vi "VDMS_NO_IEPE_FPGA_Main_6_Modules.vi"() -> ()   [LabVIEW 2017]
doc: "This VI provides a template for customizing a waveform acquisition using delta-sigma based NI C Series analog input smodules."
uses:
  <vilib>/LabVIEW Targets/FPGA/cRIO/shared/nicrio_ModuleControls/nicrio_cRIO-9232_ConfigModeRing.ctl
  <vilib>/Platform/TimedLoop/XDataNode/timing_clust.ctl
  <vilib>/Platform/TimedLoop/XDataNode/nitl_modes.ctl
  <vilib>/Platform/TimedLoop/XDataNode/wakeup.ctl
  <vilib>/rvi/Emulation/niFpgaGetClockAttributes.vi
  <vilib>/rvi/Emulation/niFpgaSctlEmulationGetInTimedLoop.vi
  <vilib>/rvi/Emulation/niFpgaEmulationReportErrorSimple.vi
  <vilib>/rvi/Emulation/niFpgaProcessEmulError.vi
  <vilib>/addons/InsightCM/Devices/Shared/Cms/Fpga/AcquisitionFpgaTach/source/subVIs/Glbl Stop.vi
  <vilib>/addons/InsightCM/Devices/Shared/Cms/Fpga/AcquisitionFpgaTach/source/subVIs/FPGA Globals.vi
  <vilib>/rvi/eio/common/nirviEmuTemplateMethod_errors.vi
  <vilib>/rvi/Memory/Memory_Emulation/nirvimemoryFastEmulation.vi
  <vilib>/rvi/Memory/Memory_Emulation/nirvimemoryEmulation.vi
  <vilib>/rvi/Emulation/niFpgaEmulationIsFPGAContextNoSignature.vi
  <vilib>/rvi/DataTransferAndStorage/Container/Common/niFpgaContainerGetUniqueNameForEmu.vi
  <vilib>/rvi/errors/nirviReportUnexpectedCaseInternalError (U32).vi
  <vilib>/rvi/DataTransferAndStorage/Container/Common/niFpgaContainerExecOnDevCompGetState.vi
  <vilib>/rvi/Memory/Memory_Emulation/niFpgaMemoryEmulationCacheClearOnFirstRun.vi
  <vilib>/rvi/Memory/Memory_Emulation/nirvimemoryEmulationManagerCache_MakeExclusive.vi
  <vilib>/rvi/Memory/Memory_Emulation/niFpgaMemoryEmulationValidateCache.vi
  <vilib>/rvi/Memory/Memory_Emulation/nirvimemoryEmulationManagerCache_InsertValue.vi
  <vilib>/Utility/error.llb/Clear Errors.vi
  <vilib>/rvi/Memory/Memory_Emulation/nirvimemoryEmulationManagerCache_ReleaseExclusive.vi
  <vilib>/rvi/Memory/Memory_Emulation/nirvimemoryEmulationManagerCache_GetValue.vi
  <vilib>/rvi/Memory/Memory_Emulation/nirvimemoryEmulationManagerCache_SetValue.vi
  <vilib>/rvi/Emulation/niFpgaSctlEmulationResourceMgr.vi
  <vilib>/rvi/Emulation/niFpgaCriticalErrorInLSC.vi
  <vilib>/rvi/interface/RandomDataEmulation/niFpgaRandomDataHandleErrors.vi
  <vilib>/rvi/errors/niFpgaSetErrorForExecOnDevCompSimple.vi
  <vilib>/rvi/eio/common/nirviEmuReportErrorAndStop.vi
  <vilib>/rvi/FIFO/Fifo_Resource/nirvififoEmulationSetSize.vi
  <vilib>/rvi/FIFO/Fifo_Resource/nirviFifoEmulationQueueMgr.vi
  <instcachedir>/0/nirviFifoEmulationQueueMgr_E5CAEC123FF24DC58D834DCA3CDAA9B5.lvgen/nirviFifoEmulationQueueMgr_E5CAEC123FF24DC58D834DCA3CDAA9B5_001.vi
  <vilib>/rvi/FIFO/Fifo_Resource/nirvififoEmulationDetermineInputValidOut.vi
  <vilib>/rvi/FIFO/Fifo_Resource/nirvififoEmulationCreateLock.vi
  <vilib>/rvi/FIFO/Fifo_Resource/nirvififoEmulationObtainLock.vi
  <vilib>/rvi/FIFO/Fifo_Resource/nirvififoEmulationReleaseLock.vi
  <vilib>/rvi/occurrence/nirviWaitOnOccurrenceBase.vi
  <vilib>/rvi/errors/nirviReportUnexpectedCaseInternalError.vi
  <vilib>/eio/EIONode/EIONode.xnode
  <vilib>/rvi/DataTransferAndStorage/Container/XNode/niFpgaContainer.xnode
  <vilib>/rvi/Memory/Memory_Emulation/niFpgaMemoryEmulationRefIn.vi
  <vilib>/Platform/TimedLoop/XDataNode/XDataNode.xnode
  <vilib>/rvi/interface/RandomDataEmulation/nirviRandomDataFpgaReadWriteTemplate.vi
  <vilib>/rvi/FXPMathLib/basic elements/FxpDiscreteDelay/XNode/nifxpmath_DiscreteDelay.xnode
  <vilib>/rvi/FIFO/Fifo_Resource/niFpgaFifoEmulationRefIn.vi
  <vilib>/addons/InsightCM/Devices/Shared/Cms/Fpga/AcquisitionFpgaTach/source/subVIs/VibAPI/VDMS_VibAPI.lvlib
  <vilib>/Platform/TimedLoop/XDataNode/XDNodeRunTimeDep.lvlib
panel:
  in  "Tach Delay":u8
  out "Chassis Temperature":sgl
  in  "Enable Chan Array":bool[](array[boolean])=[FALSE, FALSE, FALSE, FALSE, FALSE, FALSE, FALSE, FALSE, FALSE, FALSE, FALSE, FALSE, FALSE, FALSE, FALSE, FALSE, FALSE, FALSE, FALSE, FALSE, FALSE, FALSE, FALSE, FALSE]
  in  "Custom Scale Intercept":sgl[](array[numeric])=[0.0, 0.0, 0.0, 0.0, 0.0, 0.0, 0.0, 0.0, 0.0, 0.0, 0.0, 0.0, 0.0, 0.0, 0.0, 0.0, 0.0, 0.0, 0.0, 0.0, 0.0, 0.0, 0.0, 0.0]
  in  "Custom Scale Slope":sgl[](array[numeric])=[0.0, 0.0, 0.0, 0.0, 0.0, 0.0, 0.0, 0.0, 0.0, 0.0, 0.0, 0.0, 0.0, 0.0, 0.0, 0.0, 0.0, 0.0, 0.0, 0.0, 0.0, 0.0, 0.0, 0.0]
  in  "Threshold2":fxp<+/-,24,7>=-10.0
  in  "Slope2":enum16{"falling", "rising"}(ring)
  in  "Hysteresis2":fxp<+/-,24,7>=1.0
  in  "Hysteresis1":fxp<+/-,24,7>=1.0
  in  "Threshold1":fxp<+/-,24,7>=-10.0
  in  "Slope1":enum16{"falling", "rising"}(ring)
  in  "Hysteresis0":fxp<+/-,24,7>=1.0
  in  "Slope0":enum16{"falling", "rising"}(ring)
  in  "Threshold0":fxp<+/-,24,7>=-10.0
  out "Tach FIFO Full":bool
  in  "Delay Comp":u32
  out "Start Trigger":bool
  in  "Number of Modules":i16=1
  out "Open Loop Chan Array":bool[](array[boolean])
  out "Short Circuit Chan Array":bool[](array[boolean])
  in  "Input Config Array":T1[](array[typedef])=[1, 1, 1, 1, 1, 1, 1, 1, 1, 1, 1, 1, 1, 1, 1, 1, 1, 1, 1, 1, 1, 1, 1, 1] items=["AC Coupled", "DC Coupled", "IEPE AC Coupled"]
  in  "Data Rate [S/s]":u32=1280
  out "Chan Count":bool
  out "Acq Loop Ticks":u32
  out "FPGA Error":errorcluster
  out "Module Underflow":bool
  out "Finished":bool
  in  "Total Avail Channels":i32=4
  in  "Samps per Chan [Finite]":i32=5120
  out "First Read":bool
  in  "Acquisition Type":enum16{"Finite Samples", "Continuous Samples"}(ring)
  out "DMA FIFO Full":bool
  in  "Stop":bool
  # "Keyphasor Info"
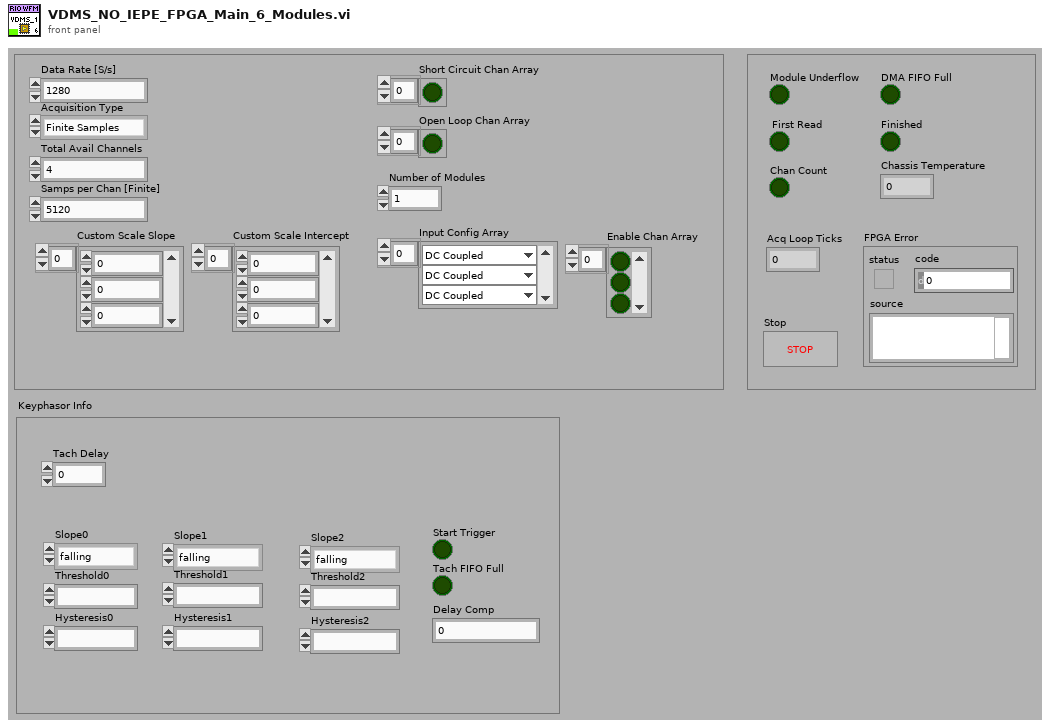
[diagram p1: front panel]
types:
  T1 = typedef "nicrio_cRIO-9232_ConfigModeRing.ctl" = u8
  T2 = typedef "XDNodeRunTimeDep.lvlib/timing_clust.ctl" = cluster{"Expected End [f-1]":u64, "Actual End [f-1]":u64, "Finished Late? [f-1]":bool, "Expected End [i-1]":u64, "Actual End [i-1]":u64, "Finished Late? [i-1]":bool, "Expected Start [i]":u64, "Actual Start [i]":u64, "Expected Start [f]":u64, "Actual Start [f]":u64, "Source Name":string, "Structure Name":string, "Period":i64, "Deadline":i64, "Offset":i64, "Start":i64, "Priority":i32, "Timeout":i32, "Mode":T3, "Wakeup Reason":T4, "Error":errorcluster, "Source Type":string, "Secondary Source Type":string, "Global End Time":u64, "Global Start Time":u64, "Frame Duration":u64, "Iteration Duration":u64, "Assigned CPU":i32, "I/O Scan Engine Mode":u32}
  T3 = typedef "XDNodeRunTimeDep.lvlib/nitl_modes.ctl" = enum32{"No Change", "Process missed periods, maintain original phase", "Discard missed periods, maintain original phase", "Process missed periods, ignore original phase", "Discard missed periods, ignore original phase"}
  T4 = typedef "XDNodeRunTimeDep.lvlib/wakeup.ctl" = enum32{"Normal", "Aborted", "Asynchronous wakeup", "Timing source error", "Timed loop error", "Timeout"}
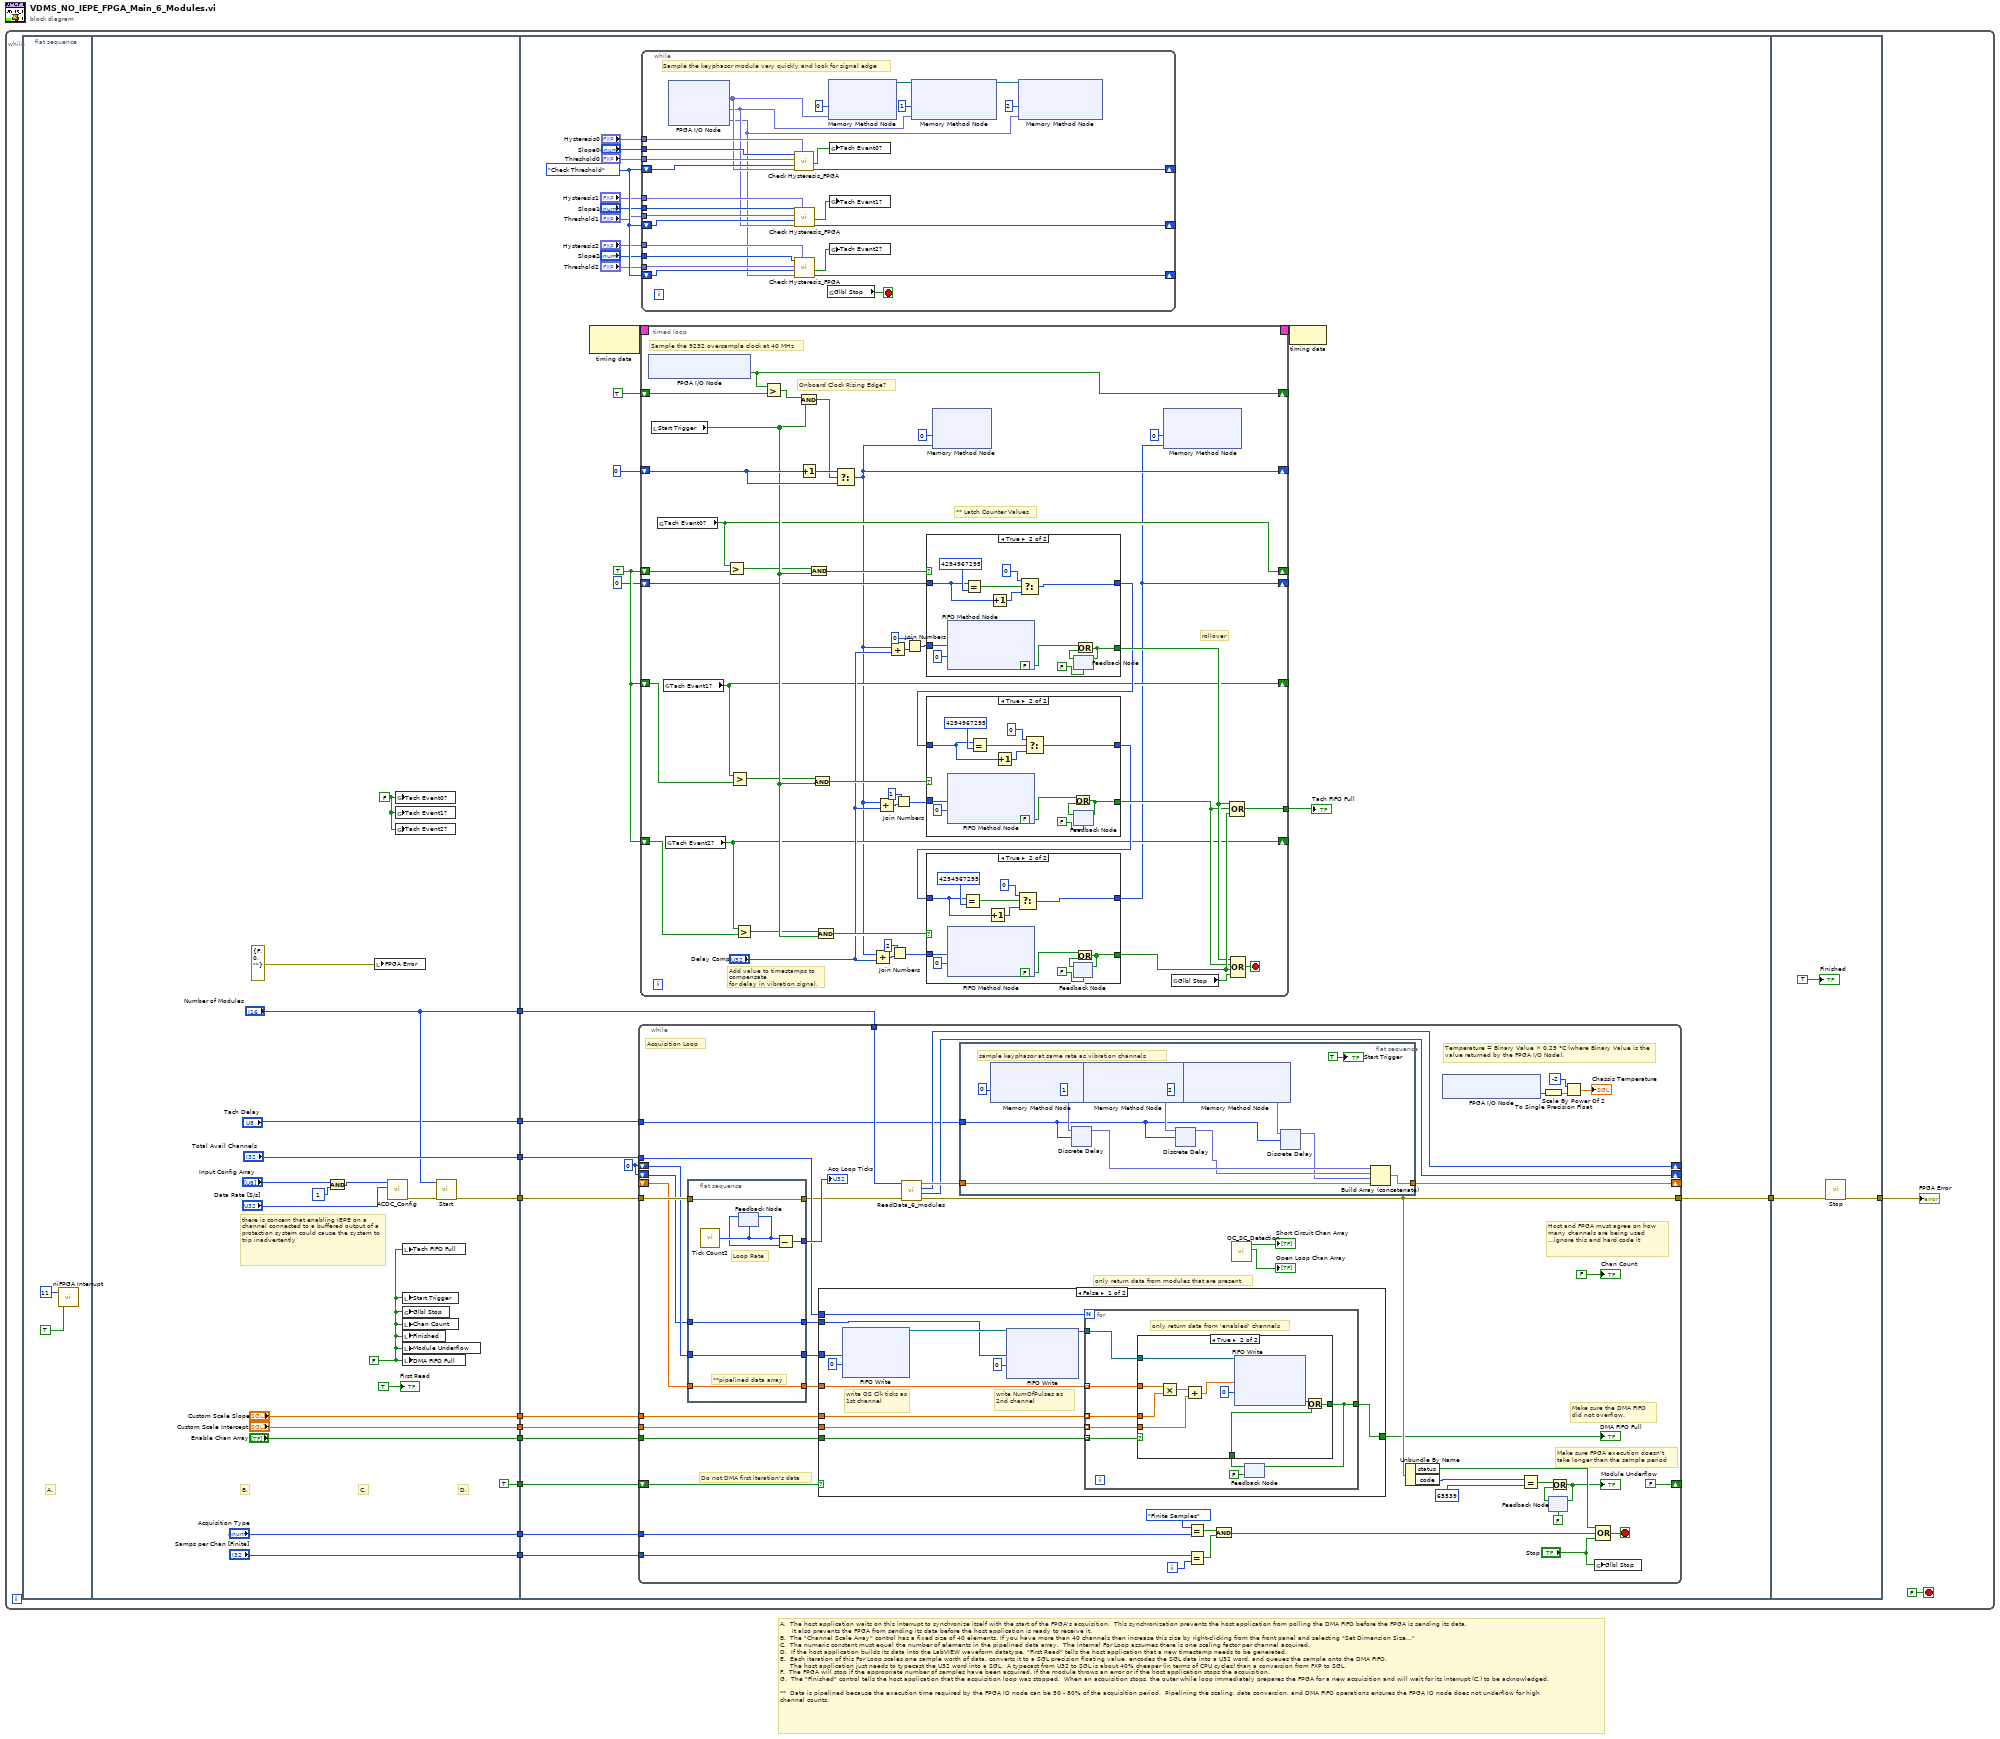
[diagram p0: block diagram]
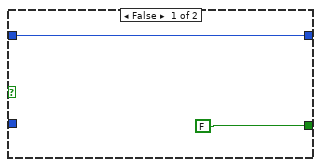
[diagram p2: hidden frame]
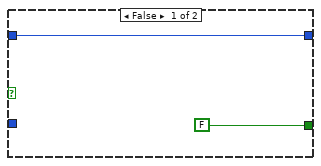
[diagram p3: hidden frame]
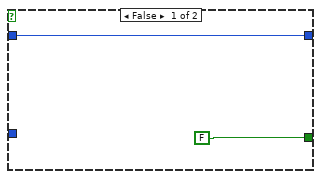
[diagram p4: hidden frame]
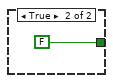
[diagram p6: hidden frame]
diagram:
  # "A.  The host application waits on this interrupt to synchronize itself with the start of the FPGA's acquisition.  This synchronization prevents the host application from polling the DMA FIFO before the FPGA is sending its data.\n      It also prevents the FPGA from sending its data before the host application is ready to receive it.\nB.  The \"Channel Scale Array\" control has a fixed size of 40 elements. If you have more than 40 channels then increase this size by right-clicking from the front panel and selecting \"Set Dimension Size...\"\nC.  The numeric constant must equal the number of elements in the pipelined data array.  The internal For Loop assumes there is one scaling factor per channel acquired.  \nD.  If the host application builds its data into the LabVIEW waveform datatype, \"First Read\" tells the host application that a new timestamp needs to be generated.\nE.  Each iteration of this For Loop scales one sample worth of data, converts it to a SGL precision floating value, encodes the SGL data into a U32 word, and queues the sample onto the DMA FIFO.  \n     The host application just needs to typecast the U32 word into a SGL.  A typecast from U32 to SGL is about 40% cheaper (in terms of CPU cycles) than a conversion from FXP to SGL.\nF.  The FPGA will stop if the appropriate number of samples have been acquired, if the module throws an error or if the host application stops the acquisition.  \nG.  The \"Finished\" control tells the host application that the acquisition loop was stopped.  When an acquisition stops, the outer while loop immediately prepares the FPGA for a new acquisition and will wait for its interrupt (C.) to be acknowledged.\n\n**  Data is pipelined because the execution time required by the FPGA IO node can be 50 - 80% of the acquisition period.  Pipelining the scaling, data conversion, and DMA FIFO operations ensures the FPGA IO node does not underflow for high\nchannel counts."
  n1 = while {
    stop <- FALSE stop-if-true
    n2 = flat-sequence {
      tunnel: [w28] -> w12
      tunnel: ["Acquisition Type"] -> w11
      tunnel: ["Samps per Chan [Finite]"] -> w10
      tunnel: ["Total Avail Channels"] -> w9
      tunnel: [TRUE ("t")] -> w8
      tunnel: ["Number of Modules"] -> w6
      tunnel: ["Custom Scale Slope"] -> w4
      tunnel: ["Custom Scale Intercept"] -> w3
      tunnel: ["Enable Chan Array"] -> w2
      tunnel: ["Tach Delay"] -> w1
      tunnel: w12 -> [w62]
      tunnel: w11 -> [w60]
      tunnel: w10 -> [w59]
      tunnel: w9 -> [w63]
      tunnel: w8 -> [w61]
      tunnel: [w58] -> w7
      tunnel: w6 -> [w57]
      tunnel: w4 -> [w40]
      tunnel: w3 -> [w39]
      tunnel: w2 -> [w38]
      tunnel: w1 -> [w35]
      tunnel: w7 -> [w280]
      tunnel: [w279] -> w5
      frame #0 {
        # "A."
        n3 = call <vilib>:"niFPGA Interrupt.vi"("Wait Until Cleared (F)"=TRUE ("Wait Until Cleared"), "IRQ Number (0)"=u8 11 ("IRQ Number")) -> ()  [unwired: 1 in]
      }
      frame #1 {
        w20 = FALSE ("Tach Event0?")
        w24 = FALSE ("Module Underflow")
        # "there is concern that enabling IEPE on a channel connected to a buffered output of a protection system could cause the system to trip inadvertently"
        # "D."
        # "C."
        # "B."
        n4 = And(x="Input Config Array", y=u8 1) -> (x .and. y?=w16:T1[])
        n5 = local write "FPGA Error"(errorcluster {"status"=FALSE, "code"=0, "source"=""} ("FPGA Error")) -> ()
        n6 = call <vilib>:"ACDC_Config.vi"("Data Rate [S/s]"="Data Rate [S/s]", "Input Config Array"=w16) -> ("error out"=w27:errorcluster)  [unwired: 9 in]
        n7 = global write "FPGA Globals.vi" "Tach Event0?"(w20) -> ()
        n8 = global write "FPGA Globals.vi" "Tach Event1?"(w20) -> ()
        n9 = global write "FPGA Globals.vi" "Tach Event2?"(w20) -> ()
        n10 = local write "Tach FIFO Full"(w24) -> ()
        n11 = local write "Start Trigger"(w24) -> ()
        n12 = global write "Glbl Stop.vi" "Glbl Stop"(w24) -> ()
        n13 = local write "Chan Count"(w24) -> ()
        n14 = local write "Finished"(w24) -> ()
        n15 = local write "Module Underflow"(w24) -> ()
        n16 = local write "DMA FIFO Full"(w24) -> ()
        n17 = call <vilib>:"Start.vi"("error in (no error)"=w27, "Module Config Selector"="Number of Modules") -> ("error out"=w28:errorcluster)  [unwired: 9 in]
        "First Read" <- TRUE ("First Read")
      }
      frame #2 {
        w36 = u32 0 ("OversampleClk Ticks")
        w48 = enum16{"Check Hysteresis", "Check Threshold"}."Check Threshold" ("State Out")
        w52 = TRUE
        n18 = node-c288() -> (w56:T2)  [unwired: 1 out]
        n19 = while {
          tunnel: w62 -> [w216]
          tunnel: [w218] -> w58
          tunnel: w60 -> [w220]
          tunnel: w59 -> [w219]
          shift-right: [w193] -> _
          shift-left: _ -> [w213]
          tunnel: w63 -> [w199]
          shift-right: [FALSE ("t")] -> _
          shift-left: w61 -> [w212]
          tunnel: w57 -> [w200]
          shift-right: [w192] -> _
          shift-left: w36 -> [w191]
          tunnel: w40 -> [w189]
          tunnel: w39 -> [w188]
          tunnel: w38 -> [w187]
          shift-right: [w186] -> _
          shift-left: w36 -> [w185]
          tunnel: w35 -> [w179]
          i -> [w210]
          stop <- w223 stop-if-true
          # "Temperature = Binary Value × 0.25 °C (where Binary Value is the value returned by the FPGA I/O Node)."
          # "only return data from modules that are present"
          # "Do not DMA first iteration's data"
          # "Acquisition Loop"
          # "Host and FPGA must agree on how \nmany channels are being used\n...ignore this and hard code it"
          # "Make sure the DMA FIFO\ndid not overflow."
          # "Make sure FPGA execution doesn't\ntake longer than the sample period"
          n20 = flat-sequence {
            tunnel: w216 -> [w274]
            tunnel: [w276] -> w215
            tunnel: w213 -> [w275]
            tunnel: [w275] -> w214
            tunnel: [w274] -> w195
            tunnel: [w273] -> w190
            tunnel: w191 -> [w273]
            tunnel: [w272] -> w184
            tunnel: w185 -> [w272]
            frame #0 {
              # "**pipelined data array"
              # "Loop Rate"
              n21 = call "Tick Count2"() -> ("Tick Count(Ticks)"=w278:u32)
              n22 = feedback-in #1(w278) -> ()
              n23 = feedback #1(w278) -> (w277:u32)
              n24 = Subtract(x=w278, y=w277) -> (x-y=w276:u32)
            }
          }
          n25 = case shown="False" w212 {
            tunnel: [w244 FALSE] -> w217
            tunnel: w214 -> [w248 _]
            tunnel: w199 -> [w249 _]
            tunnel: w190 -> [w250 _]
            tunnel: w189 -> [w247 _]
            tunnel: w188 -> [w246 _]
            tunnel: w187 -> [w245 _]
            tunnel: w184 -> [w240 _]
            frame False {
              # "write NumOfPulses as 2nd channel"
              # "write OS Clk ticks as 1st channel"
              n26 = xnode ("FIFO Write")("Element"=w250, "Timeout"=0) -> ("FIFO Out"=w243:refnum<k21>)  [unwired: 1 in, 1 out]
              n27 = xnode ("FIFO Write")("Element"=w240, "Timeout"=0, "FIFO In"=w243) -> ("FIFO Out"=w241:refnum<k21>)  [unwired: 1 out]
              n28 = for {
                N: w249 -> [_]
                tunnel: [w258] -> w244
                tunnel: w248 -> [w257] mode=indexing
                tunnel: w247 -> [w256] mode=indexing
                tunnel: w245 -> [w254] mode=indexing
                tunnel: w246 -> [w253] mode=indexing
                tunnel: w241 -> [w252]
                # "only return data from 'enabled' channels"
                n29 = feedback #2(FALSE) -> (w259:bool)
                n30 = case shown="True" w254 {
                  tunnel: w259 -> [w260 w270]
                  tunnel: [w260 w269] -> w258
                  tunnel: w257 -> [_ w268]
                  tunnel: w256 -> [_ w267]
                  tunnel: w253 -> [_ w262]
                  tunnel: w252 -> [_ w261]
                  frame False {
                  }
                  frame True {
                    n31 = Multiply(x=w268, y=w267) -> (x*y=w264:sgl)
                    n32 = Add(x=w264, y=w262) -> (x+y=w263:sgl)
                    n33 = xnode ("FIFO Write")("Element"=w263, "Timeout"=0, "FIFO In"=w261) -> ("Timed Out?"=w265:bool)  [unwired: 1 out]
                    n34 = Or(x=w265, y=w270) -> (x .or. y?=w269:bool)
                  }
                }
                n35 = feedback-in #2(w258) -> ()
              }
            }
            frame True {
            }
          }
          "DMA FIFO Full" <- w217
          n36 = call <vilib>:"ReadData_6_modules.vi"("error in"=w195, "Module Config Selector"=w200) -> ("error out"=w218:errorcluster, "Number Of Pulses"=w186:u32, "OversampleClk Ticks"=w192:u32, "Data Array"=w194:sgl[])  [unwired: 6 in]
          n37 = flat-sequence {
            tunnel: w194 -> [w239]
            tunnel: [w238] -> w193
            tunnel: w179 -> [w225]
            frame #0 {
              # "sample keyphasor at same rate as vibration channels"
              n38 = xnode ("Memory Method Node")("Address"=u32 0) -> ("Data"=w231:fxp<+/-,24,7>, "Memory Out"=w235:refnum<k21>)  [unwired: 1 in]
              n39 = xnode ("Discrete Delay")("D"=w231, "n-1[0..31]"=w225) -> ("Q"=w230:fxp<+/-,24,7>)
              n40 = xnode ("Memory Method Node")("Address"=u32 1, "Memory In"=w235) -> ("Data"=w229:fxp<+/-,24,7>, "Memory Out"=w234:refnum<k21>)
              n41 = xnode ("Discrete Delay")("D"=w229, "n-1[0..31]"=w225) -> ("Q"=w228:fxp<+/-,24,7>)
              n42 = xnode ("Memory Method Node")("Address"=u32 2, "Memory In"=w234) -> ("Data"=w227:fxp<+/-,24,7>)  [unwired: 1 out]
              n43 = xnode ("Discrete Delay")("D"=w227, "n-1[0..31]"=w225) -> ("Q"=w226:fxp<+/-,24,7>)
              n44 = Build Array (concatenate)(w230, w228, w226, w239) -> (w238:sgl[])
              "Start Trigger" <- TRUE ("Start Trigger")
            }
          }
          n45 = Equal?(x=enum16{"Finite Samples", "Continuous Samples"}."Finite Samples" ("y"), y=w220) -> (x = y?=w204:bool)
          n46 = Equal?(x=w219, y=w210) -> (x = y?=w203:bool)
          n47 = And(x=w204, y=w203) -> (x .and. y?=w202:bool)
          n48 = call <vilib>:"OC_SC_Detection.vi"() -> ("Open Loop Channels Array"=→"Open Loop Chan Array":bool[], "Short Circuit Channels Array"=→"Short Circuit Chan Array":bool[])  [unwired: 10 in]
          n49 = Unbundle By Name(w218) -> ("status"=w209:bool, "code"=w221:i32)
          n50 = xnode "FPGA I/O Node"() -> ("Chassis Temperature"=w181:i16)  [unwired: 1 in, 1 out]
          n51 = Equal?(x=w221, y=65539) -> (x = y?=w206:bool)
          n52 = To Single Precision Float(number=w181) -> (single precision float=w183:sgl)
          n53 = feedback #3(FALSE) -> (w208:bool)
          n54 = Or(x=w206, y=w208) -> (x .or. y?=w205:bool)
          "Module Underflow" <- w205
          n55 = feedback-in #3(w205) -> ()
          n56 = Scale By Power Of 2(n=i16 -2, x=w183) -> (x*2^n=→"Chassis Temperature":sgl)
          n57 = global write "Glbl Stop.vi" "Glbl Stop"("Stop") -> ()
          n58 = Compound Arithmetic op=OR(w209, w202, "Stop") -> (w223:bool)
          "Chan Count" <- FALSE ("Chan Count")
          "Acq Loop Ticks" <- w215
        }
        n59 = timed-loop {
          timing: w56 -> [_]
          timing-out: [_] -> w55
          shift-right: [w94] -> _
          shift-left: u32 0 -> [w129]
          shift-right: [w131] -> _
          shift-left: TRUE -> [w132]
          shift-right: [w97] -> _
          shift-left: w52 -> [w128]
          shift-right: [w96] -> _
          shift-left: w52 -> [w122]
          shift-right: [w95] -> _
          shift-left: w52 -> [w121]
          tunnel: [w103] -> w41
          shift-right: [w93] -> _
          shift-left: u32 0 -> [w100]
          stop <- w127 stop-if-true
          # "rollover"
          # "** Latch Counter Values"
          # "Add value to timestamps to compensate \nfor delay in vibration signal."
          # "Sample the 9232 oversample clock at 40 MHz"
          # "Onboard Clock Rising Edge?"
          n60 = xnode "FPGA I/O Node"() -> ("Mod1/Onboard Clock"=w131:bool)  [unwired: 1 in, 1 out]
          n61 = local read "Start Trigger"() -> (w120:bool)
          n62 = global read "FPGA Globals.vi" "Tach Event0?"() -> (w97:bool)
          n63 = global read "FPGA Globals.vi" "Tach Event1?"() -> (w96:bool)
          n64 = global read "FPGA Globals.vi" "Tach Event2?"() -> (w95:bool)
          n65 = Greater?(x=w97, y=w128) -> (0:w119:bool)
          n66 = Greater?(x=w96, y=w122) -> (0:w118:bool)
          n67 = Greater?(x=w95, y=w121) -> (0:w117:bool)
          n68 = Greater?(x=w131, y=w132) -> (0:w126:bool)
          n69 = And(x=w126, y=w120) -> (x .and. y?=w125:bool)
          n70 = Increment(x=w129) -> (x+1=w130:u32)
          n71 = And(x=w119, y=w120) -> (x .and. y?=w116:bool)
          n72 = And(x=w118, y=w120) -> (x .and. y?=w114:bool)
          n73 = And(x=w117, y=w120) -> (x .and. y?=w108:bool)
          n74 = Select(t=w130, s=w125, f=w129) -> (s? t:f=w94:u32)
          n75 = Add(x=w94, y="Delay Comp") -> (x+y=w110:u32)
          n76 = Add(x=w94, y="Delay Comp") -> (x+y=w113:u32)
          n77 = Add(x=w94, y="Delay Comp") -> (x+y=w124:u32)
          n78 = Join Numbers(hi=u32 2, lo=w110) -> ((hi.lo)=w106:u64)
          n79 = Join Numbers(hi=u32 1, lo=w113) -> ((hi.lo)=w111:u64)
          n80 = Join Numbers(hi=u32 0, lo=w124) -> ((hi.lo)=w123:u64)
          n81 = case shown="True" w116 {
            tunnel: [FALSE w173] -> w102
            tunnel: w123 -> [_ w170]
            tunnel: w100 -> [w161 w166]
            tunnel: [w161 w163] -> w99
            frame False {
            }
            frame True {
              (unwired) FALSE
              n82 = xnode ("FIFO Method Node")("Element"=w170, "Timeout"=0) -> ("Timed Out?"=w171:bool)  [unwired: 1 in, 1 out]
              n83 = Equal?(x=w166, y=u32 4294967295) -> (x = y?=w167:bool)
              n84 = Increment(x=w166) -> (x+1=w165:u32)
              n85 = Select(t=u32 0, s=w167, f=w165) -> (s? t:f=w163:u32)
              n86 = feedback #4(FALSE) -> (w174:bool)
              n87 = Or(x=w171, y=w174) -> (x .or. y?=w173:bool)
              n88 = feedback-in #4(w173) -> ()
            }
          }
          n89 = case shown="True" w114 {
            tunnel: [FALSE w159] -> w101
            tunnel: w111 -> [_ w156]
            tunnel: w99 -> [w147 w150]
            tunnel: [w147 w149] -> w98
            frame False {
            }
            frame True {
              (unwired) FALSE
              n90 = xnode ("FIFO Method Node")("Element"=w156, "Timeout"=0) -> ("Timed Out?"=w157:bool)  [unwired: 1 in, 1 out]
              n91 = Equal?(x=w150, y=u32 4294967295) -> (x = y?=w152:bool)
              n92 = Increment(x=w150) -> (x+1=w153:u32)
              n93 = Select(t=u32 0, s=w152, f=w153) -> (s? t:f=w149:u32)
              n94 = feedback #5(FALSE) -> (w160:bool)
              n95 = Or(x=w157, y=w160) -> (x .or. y?=w159:bool)
              n96 = feedback-in #5(w159) -> ()
            }
          }
          n97 = case shown="True" w108 {
            tunnel: [FALSE w145] -> w104
            tunnel: w106 -> [_ w142]
            tunnel: w98 -> [w133 w136]
            tunnel: [w133 w135] -> w93
            frame False {
            }
            frame True {
              (unwired) FALSE
              n98 = xnode ("FIFO Method Node")("Element"=w142, "Timeout"=0) -> ("Timed Out?"=w143:bool)  [unwired: 1 in, 1 out]
              n99 = Equal?(x=w136, y=u32 4294967295) -> (x = y?=w139:bool)
              n100 = Increment(x=w136) -> (x+1=w138:u32)
              n101 = Select(t=u32 0, s=w139, f=w138) -> (s? t:f=w135:u32)
              n102 = feedback #6(FALSE) -> (w146:bool)
              n103 = Or(x=w143, y=w146) -> (x .or. y?=w145:bool)
              n104 = feedback-in #6(w145) -> ()
            }
          }
          n105 = xnode ("Memory Method Node")("Address"=u32 0, "Data"=w94) -> ()  [unwired: 1 in, 1 out]
          n106 = xnode ("Memory Method Node")("Address"=u32 0, "Data"=w93) -> ()  [unwired: 1 in, 1 out]
          n107 = global read "Glbl Stop.vi" "Glbl Stop"() -> (w105:bool)
          n108 = Compound Arithmetic op=OR(w102, w101, w104) -> (w103:bool)
          n109 = Compound Arithmetic op=OR(w102, w101, w104, w105) -> (w127:bool)
        }
        "Tach FIFO Full" <- w41
        n110 = while {
          shift-right: [w88] -> _
          shift-left: w48 -> [w89]
          tunnel: "Slope0" -> [w87]
          tunnel: "Threshold0" -> [w86]
          tunnel: "Hysteresis0" -> [w85]
          shift-right: [w84] -> _
          shift-left: w48 -> [w82]
          shift-right: [w83] -> _
          shift-left: w48 -> [w81]
          tunnel: "Hysteresis1" -> [w80]
          tunnel: "Slope1" -> [w79]
          tunnel: "Threshold1" -> [w78]
          tunnel: "Hysteresis2" -> [w77]
          tunnel: "Slope2" -> [w76]
          tunnel: "Threshold2" -> [w75]
          stop <- w90 stop-if-true
          # "Sample the keyphasor module very quickly and look for signal edge"
          n111 = xnode "FPGA I/O Node"() -> ("Mod1/AI0"=w66:fxp<+/-,24,7>, "Mod1/AI1"=w65:fxp<+/-,24,7>, "Mod1/AI2"=w64:fxp<+/-,24,7>)  [unwired: 3 in, 3 out]
          n112 = call <vilib>:"Check Hysteresis_FPGA.vi"("Hysteresis"=w85, "Analog In (Tach)"=w66, "State In"=w89, "Threshold"=w86, "Slope"=w87) -> ("State Out"=w88:enum16{"Check Hysteresis", "Check Threshold"}, "Event Ocurred?"=w73:bool)  [unwired: 2 in]
          n113 = call <vilib>:"Check Hysteresis_FPGA.vi"("Hysteresis"=w80, "Analog In (Tach)"=w65, "State In"=w82, "Threshold"=w78, "Slope"=w79) -> ("State Out"=w84:enum16{"Check Hysteresis", "Check Threshold"}, "Event Ocurred?"=w74:bool)  [unwired: 2 in]
          n114 = call <vilib>:"Check Hysteresis_FPGA.vi"("Hysteresis"=w77, "Analog In (Tach)"=w64, "State In"=w81, "Threshold"=w75, "Slope"=w76) -> ("State Out"=w83:enum16{"Check Hysteresis", "Check Threshold"}, "Event Ocurred?"=w72:bool)  [unwired: 2 in]
          n115 = global read "Glbl Stop.vi" "Glbl Stop"() -> (w90:bool)
          n116 = xnode ("Memory Method Node")("Address"=u32 0, "Data"=w66) -> ("Memory Out"=w68:refnum<k21>)  [unwired: 1 in]
          n117 = global write "FPGA Globals.vi" "Tach Event0?"(w73) -> ()
          n118 = global write "FPGA Globals.vi" "Tach Event1?"(w74) -> ()
          n119 = global write "FPGA Globals.vi" "Tach Event2?"(w72) -> ()
          n120 = xnode ("Memory Method Node")("Address"=u32 1, "Data"=w65, "Memory In"=w68) -> ("Memory Out"=w69:refnum<k21>)
          n121 = xnode ("Memory Method Node")("Address"=u32 2, "Data"=w64, "Memory In"=w69) -> ()  [unwired: 1 out]
        }
        n122 = node-c288(w55) -> ()
      }
      frame #3 {
        n123 = call <vilib>:"Stop.vi"("error in (no error)"=w280) -> ("error out"=w279:errorcluster)  [unwired: 10 in]
        "Finished" <- TRUE ("Finished")
      }
    }
    "FPGA Error" <- w5
  }
